vi "CalcExtension.vi"(8 "Offset":dbl, 9 "AOM X Cal":dbl, 10 "Trap Positions":waveform(dbl)[](array[waveform]), 11 "BeadDeflection":waveform(dbl)) -> (3 "Extension":waveform(dbl))   [LabVIEW 2013]
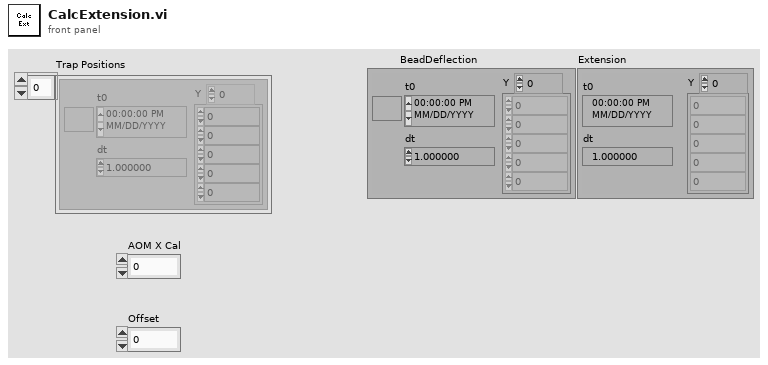
[diagram p1: front panel]
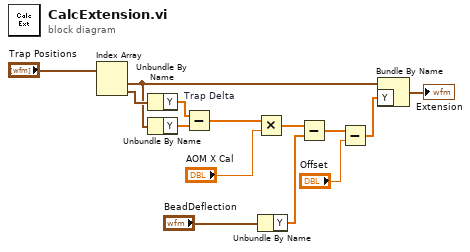
[diagram p0: block diagram]
diagram:
  n1 = Index Array(array="Trap Positions") -> (element #1=w2:waveform(dbl), element #2=w6:waveform(dbl))  [unwired: 2 in]
  n2 = Unbundle By Name(w6) -> ("Y"=w5:dbl[])
  n3 = Unbundle By Name(w2) -> ("Y"=w4:dbl[])
  n4 = Subtract "Trap Delta"(x=w5, y=w4) -> (x-y=w3:dbl[])
  n5 = Multiply(x=w3, y="AOM X Cal") -> (x*y=w12:dbl[])
  n6 = Unbundle By Name("BeadDeflection") -> ("Y"=w11:dbl[])
  n7 = Subtract(x=w12, y=w11) -> (x-y=w8:dbl[])
  n8 = Subtract(x=w8, y="Offset") -> (x-y=w7:dbl[])
  n9 = Bundle By Name(cluster=w2, "Y"=w7) -> (→"Extension":waveform(dbl))
